vi "Parse State Queue++.vi"(0 "State Queue":string, 1 "Name(\"\" to use uuid)":string, 2 "Response Arguments":string, 7 "Error In (no error)":errorcluster, 9 "Dequeue Timeout(0ms)":i32, 11 "Response Timeout(5000ms)":i32=5000) -> (3 "Name Used":string, 4 "Remaining States":string, 6 "Current State":string, 8 "Arguments":string, 10 "Argument - State":string, 15 "From Who":string)   [LabVIEW 2014, in "JKI State Machine++.lvlib"]
doc: "Parses the JKI State Machine state queue and returns the current state that will execute next with the associated arguments.\n\n\n<b>Inputs:</b>\n - <b>State Queue</b>: The entire state queue is wired to this input. This should come from the main JKI State Machine shift register.\n - <b>Error In (no error)</b>: The error cluster from the JKI State Machine is wired to this input. If an error occures and appears on this input, the current state output returns the \"Error Handler\" state.\n - <b>Name(\"\" to use uuid)</b>: Module Name\n - If Input is \"\", an uuid will be used for module name. The module is marked as stand-alone mode and will not be included in module list.\n - Fi Input end with '#', the module will worked in worker mode. Modules with the same name will shared the same message queue. Any external message will be processed by one of the modules, depends on who is free.\n - Otherwise, the input string will be used as module name, which should be unique in system. JKISM will go to \"Critical Error\" state if duplicated module name is used in system.\n - <b>Response Timeout(5000ms)</b>: The timeout of waiting for response of sync-call from outside.\n - <b>Dequeue Timeout(0ms)</b>: The timeout of checking JKISM message queue.\n - <b>Response Arguments</b>: The response arguments from last state. It should come from the JKISM shift register.\n\n<b>Outputs:</b>\n - <b>Remaining States</b>: Returns all the next states that should execute after the current state completes. These should be passed through the current state in the state machine. These can also be modified or augmented within the current state if necessary.\n - <b>Arguments</b>: Returns any argument(s) that may be used in the current state string. These arguments come after the \">>\" characters. <b>Note:</b> The arguments variable must not contain any unprintable characters like linefeed or carriage return.\n - <b>Current State</b>: The state to be processed\n - <b>Name Used</b>: The actual name assigned to this JKISM module\n - <b>Argument - State</b>: If any core error occurs, this is the source state name\n - <b>From Who</b>: If <b>Current State</b> is called by ouside, this is the source JKISM module name."
uses:
  JKI State Machine++.lvlib
  _Support/Typedef/_Cross JKISM State Data.ctl
  _Support/Typedef/_JKISM_MSG_TYPE.ctl
  _Support/Typedef/_Cross JKISM State Response.ctl
  _Support/Typedef/_JKISM Status Change Event Data.ctl
  _Support/Typedef/_JKISM_GlobalLog_MSG.ctl
  _Support/Typedef/_JKISM_GlobalLog_MSG_TYPE.ctl
  _Support/JKISMQ/_Input Name to JKISM Mode.vi
  Utility/uuid.vi
  _Support/KeyWords.vi
  _Support/JKISMQ/_JKISMQFGV.vi
  _Support/FGV-BroadcastRegistry/FGV-BroadcastRegistry.vi
  _Support/FGV-BroadcastRegistry/global-Broadcast Cache Change Flag.vi
  <vilib>/regexp/Match Regular Expression.xnode
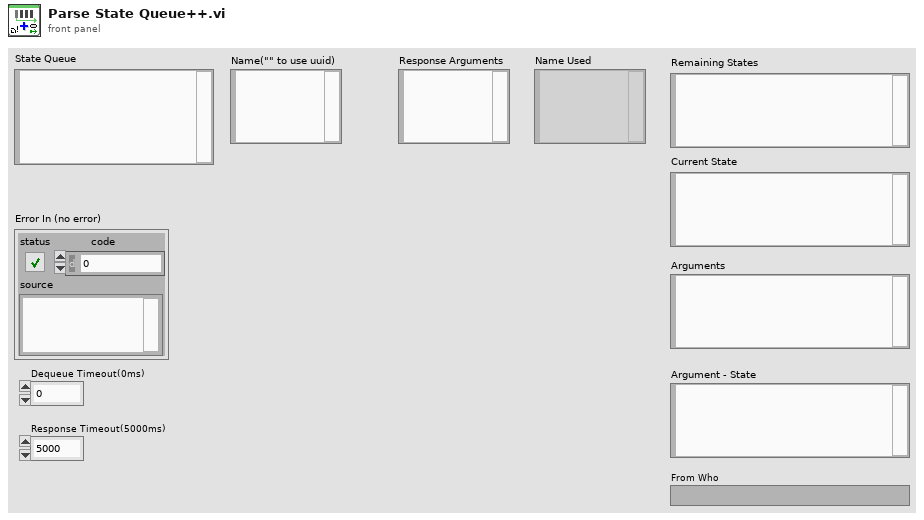
[diagram p1: front panel]
types:
  T1 = typedef "JKI State Machine++.lvlib/_JKISMQ.ctl" = cluster{"Module Name":string, "Queue":refnum<queue>, "Locked Status":refnum<data-value>, "Mode":T2, "User Event":refnum<user-event>, "Queue Count":i32, "Status Change Event":refnum<user-event>}
  T2 = typedef "JKI State Machine++.lvlib/_JKISM_MODE.ctl" = enum16{"Stand Alone", "JKISM", "Action Worker"}
  T3 = typedef "JKI State Machine++.lvlib/_JKISM_GlobalLog_MSG.ctl" = cluster{"Name(\"\" to use uuid)":string, "Current State":string, "Arguments":string, "Argument - State":string, "From Who":string, "Complete(T)/Start(F)":bool, "Type":T4}
  T4 = typedef "JKI State Machine++.lvlib/_JKISM_GlobalLog_MSG_TYPE.ctl" = enum16{"User Log", "State Change", "Status Change", "Register", "Unregister"}
  T5 = typedef "JKI State Machine++.lvlib/_JKISM_MSG_TYPE.ctl" = enum16{"Sync Message(-@)", "Async Message(->)", "Async without Response(->|)", "Async Response", "Broadcast(-><status>)", "Broadcast(-><interrupt>)", "Request to Post Message", "Request to Post Message without Reply", "Request to Publish Status"}
  T6 = typedef "JKI State Machine++.lvlib/_Cross JKISM State Data.ctl" = cluster{"Msg Type":T5, "state":string, "args":string, "source":string, "RespQ":refnum<queue>, "Pre-State":string, "Arg-State":string, "Target":string}
  T7 = typedef "JKI State Machine++.lvlib/_JKISM Status Change Event Data.ctl" = cluster{"ModuleName":string, "Status":string, "Arguments":string}
  T8 = typedef "JKI State Machine++.lvlib/_Cross JKISM State Response.ctl" = cluster{"error":errorcluster, "Response Data":string, "From Who":string}
  T9 = typedef "JKI State Machine++.lvlib/_JKISM_Broadcast_Response_Message_info.ctl" = cluster{"response message":string, "Priority":T10}
  T10 = typedef "JKI State Machine++.lvlib/JKISM++ Broadcast Message Type.ctl" = enum16{"Status", "Interrupt(High)"}
  T11 = cluster{"Target JKISM":string, "Target State":T9}[]
  T12 = typedef "JKI-State-Machine-Plus.lvlib/_Cross JKI StateMachine State Response.ctl" = cluster{"error":errorcluster, "Response Data":string, "From Who":string}
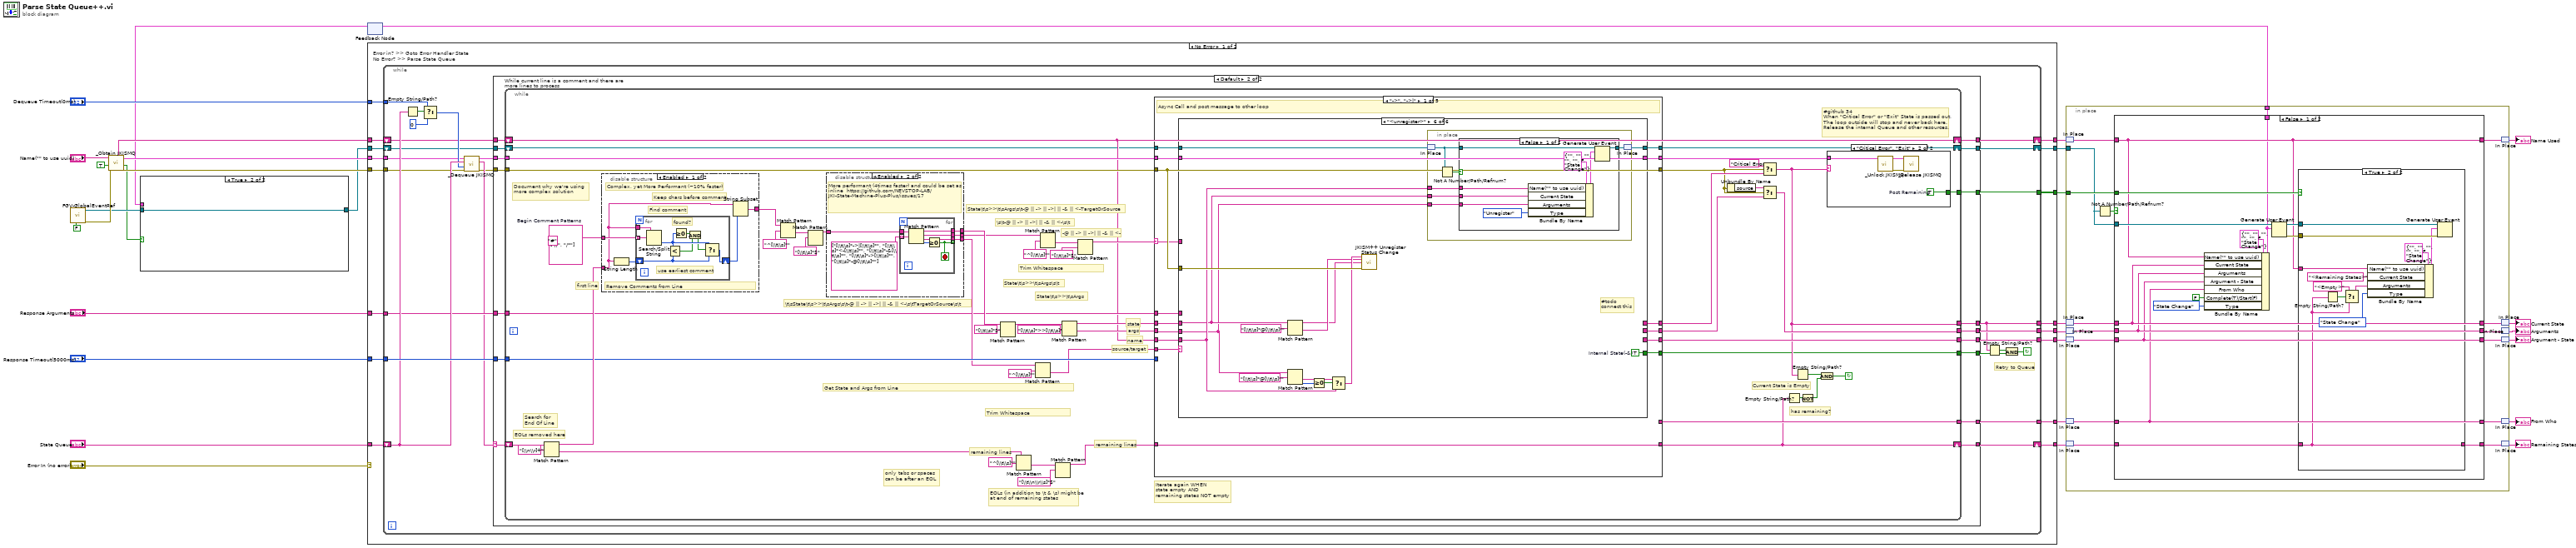
[diagram p0: block diagram]
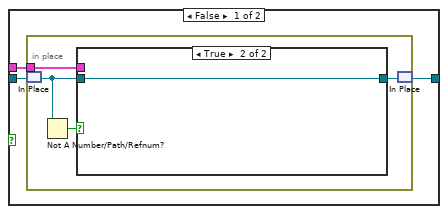
[diagram p2: hidden frame]
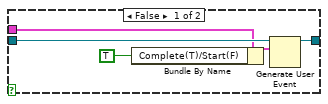
[diagram p3: hidden frame]
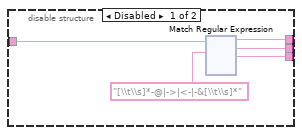
[diagram p7: hidden frame]
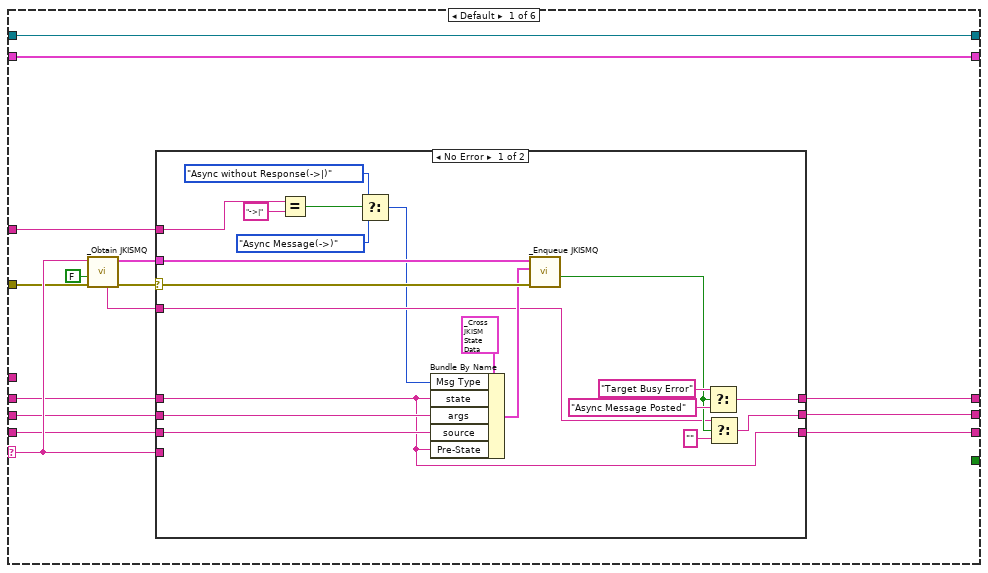
[diagram p9: hidden frame]
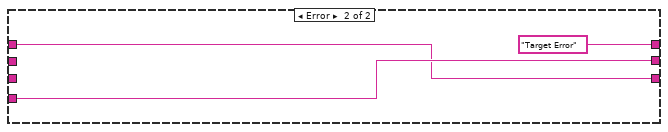
[diagram p10: hidden frame]
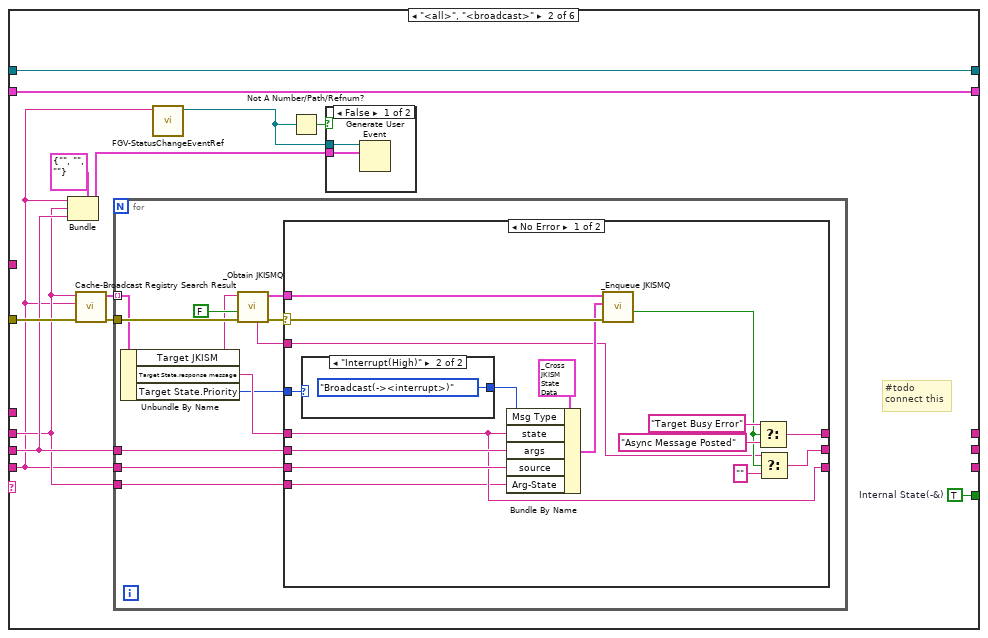
[diagram p11: hidden frame]
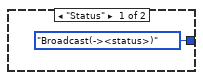
[diagram p13: hidden frame]
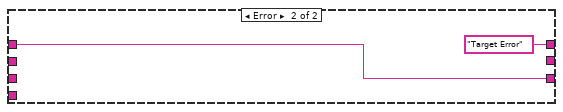
[diagram p14: hidden frame]
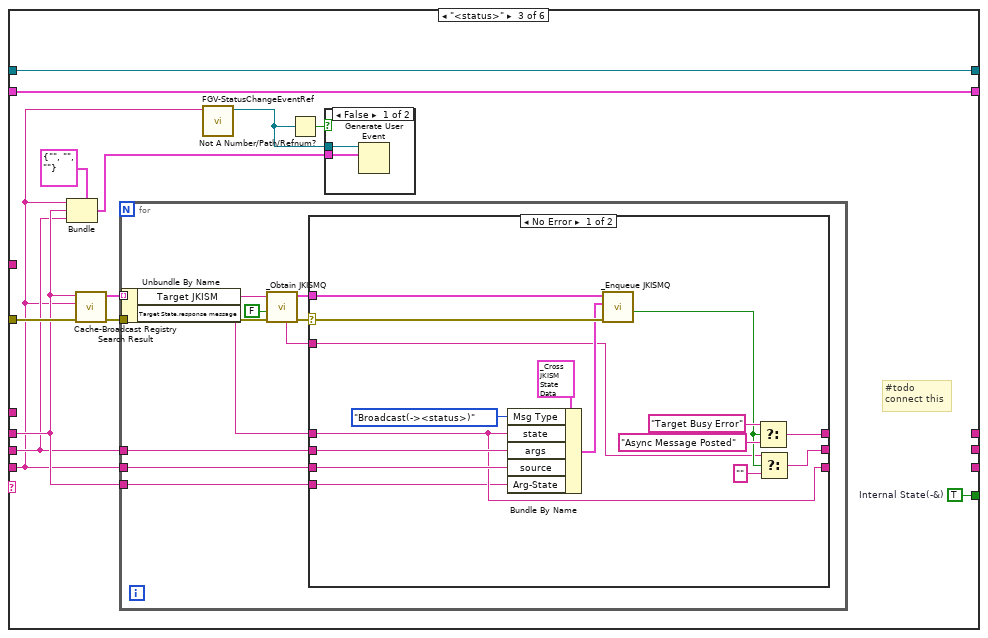
[diagram p15: hidden frame]
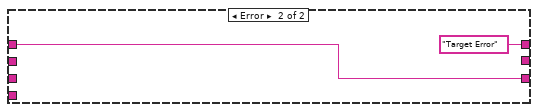
[diagram p17: hidden frame]
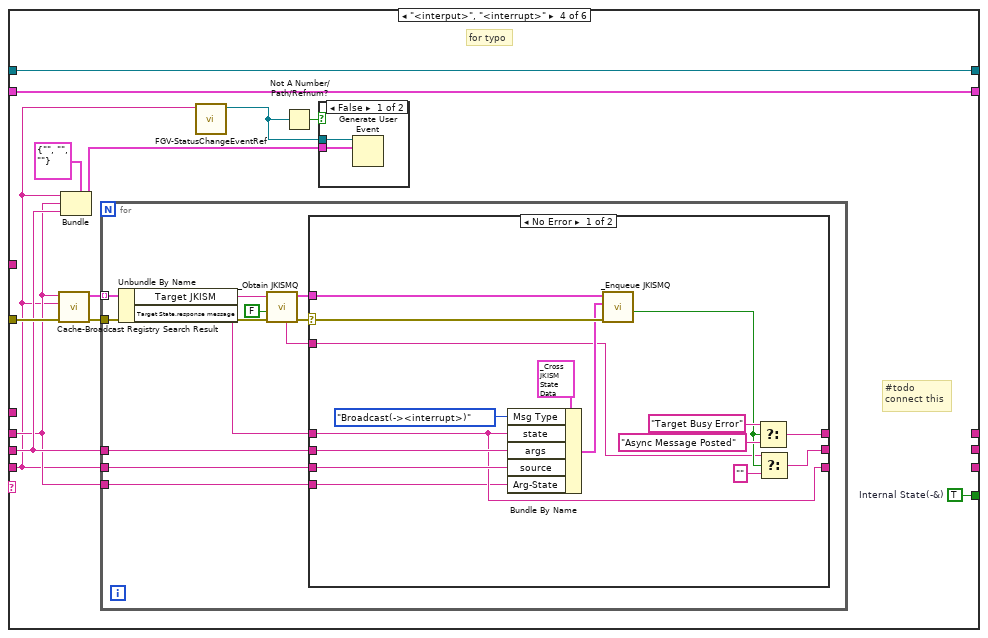
[diagram p18: hidden frame]
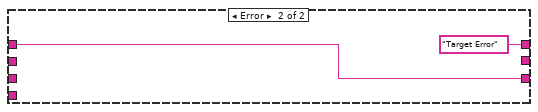
[diagram p20: hidden frame]
diagram:
  n1 = call "FGV-GlobalEventRef.vi"("Create(F)"=FALSE) -> ("error out"=w9:errorcluster, "JKISM Global Log Event"=w8:refnum<user-event>)  [unwired: 9 in]
  n2 = call "_Obtain JKISMQ.vi"("Error in"=w9, "create if not found? (T)"=TRUE, "Name(\"\" to use uuid) in"="Name(\"\" to use uuid)") -> ("Error out"=w25:errorcluster, "Create(T)/Cached(F)"=w4:bool, "JKISMQ"=w24:T1, "Name"=w3:string)  [unwired: 5 in]
  n3 = feedback #1() -> (w1:T3)  [unwired: 1 in]
  n4 = case shown="True" w4 {
    tunnel: w8 -> [w34 w45]
    tunnel: [w33 w45] -> w7
    tunnel: w1 -> [w32 _]
    frame False {
      n5 = in-place {
        in-place-border: w32 -> [w35]
        n6 = in-place-match #2(w34) -> (w37:refnum<user-event>)
        n7 = Not A Number/Path/Refnum?(number/path/refnum=w37) -> (NaN/Path/Refnum?=w38:bool)
        n8 = case shown="True" w38 {
          tunnel: w37 -> [w43 w44]
          tunnel: [w40 w44] -> w36
          tunnel: w35 -> [w39 _]
          frame False {
            n9 = Bundle By Name(cluster=w39, "Complete(T)/Start(F)"=TRUE) -> (w42:T3)
            n10 = Generate User Event(user event=w43, event data cluster=w42) -> (user event out=w40:refnum<user-event>)  [unwired: 2 in, 1 out]
          }
          frame True {
          }
        }
        n11 = in-place-match #2(w36) -> (w33:refnum<user-event>)
      }
    }
    frame True {
    }
  }
  n12 = case "Error in? >> Goto Error Handler State\nNo Error? >> Parse State Queue" shown="No Error" "Error In (no error)" {
    selector: "Error In (no error)" -> [_ w763]
    tunnel: [w59 w765] -> w13
    tunnel: [w61 "Error Handler"] -> w23
    tunnel: [w60 w759] -> w22
    tunnel: "State Queue" -> [w56 w765]
    tunnel: "Response Timeout(5000ms)" -> [w58 _]
    tunnel: w24 -> [w51 _]
    tunnel: [w57 _] -> w20
    tunnel: "Dequeue Timeout(0ms)" -> [w55 _]
    tunnel: [w54 _] -> w21
    tunnel: "Response Arguments" -> [w53 _]
    tunnel: w25 -> [w52 _]
    tunnel: w3 -> [w50 w757]
    tunnel: [w49 _] -> w14
    tunnel: w7 -> [w48 w756]
    tunnel: [w47 w757] -> w6
    tunnel: [w46 w756] -> w5
    frame No Error {
      n13 = while {
        tunnel: [w86] -> w60
        tunnel: w58 -> [w84]
        tunnel: [w83] -> w57
        tunnel: w55 -> [w79]
        tunnel: w52 -> [w74]
        tunnel: w51 -> [w73]
        shift-right: [w85] -> w59
        shift-left: w56 -> [w80]
        tunnel: w53 -> [w75]
        tunnel: [w67] -> w61
        tunnel: [w76] -> w54
        tunnel: [w65] -> w49
        shift-right: [w63] -> w47
        shift-left: w50 -> [w72]
        shift-right: [w62] -> w46
        shift-left: w48 -> [w64]
        stop <- w69 continue-if-true
        # "Retry to Queue"
        n14 = Empty String/Path?(string/path=w80) -> (empty?=w81:bool)
        n15 = Select(t=w79, s=w81, f=0) -> (s? t:f=w77:i32)
        n16 = call "_Dequeue JKISMQ.vi"("Error in"=w74, "Dequeue Timeout(0ms)"=w77, "State(s) in (\"\")"=w80, "JKISMQ in"=w73) -> ("Error out"=w70:errorcluster, "States Out"=w71:string, "JKISMQ out"=w82:T1)  [unwired: 5 in]
        n17 = case shown="Default" w71 {
          selector: w71 -> [_ w98]
          tunnel: [_ w104] -> w67
          tunnel: [_ w103] -> w86
          tunnel: [_ w102] -> w85
          tunnel: w84 -> [_ w101]
          tunnel: [_ w100] -> w83
          tunnel: w72 -> [w88 w99]
          tunnel: w82 -> [_ w97]
          tunnel: w70 -> [_ w96]
          tunnel: [_ w95] -> w76
          tunnel: w75 -> [_ w94]
          tunnel: [_ w93] -> w68
          tunnel: [_ w92] -> w65
          tunnel: w64 -> [w87 w91]
          tunnel: [w88 w90] -> w63
          tunnel: [w87 w89] -> w62
          frame "" {
            # "Dispatch Mode\n1. Error will Occurred\n2. Add Macro: Exit\n3. The Queue will regenerated\n4. But it will go Through Macro: Exit\n5. After Exit(queue released), then another Worker will be triggered."
            # "Do Nothing if Empty String"
            # "<< Wiring into the Case Selector is much more performant than using \"Empty String/Path?\" primitive"
          }
          frame Default {
            n18 = while "While current line is a comment and there are more lines to process" {
              tunnel: [w115] -> w104
              tunnel: [w119] -> w103
              shift-right: [w108] -> w102
              shift-left: w98 -> [w153]
              tunnel: w101 -> [w147]
              tunnel: [w118] -> w100
              tunnel: w97 -> [w146]
              tunnel: w96 -> [w123]
              tunnel: [w125] -> w95
              tunnel: w94 -> [w124]
              tunnel: [w112] -> w93
              tunnel: [w110] -> w92
              shift-right: [w107] -> w90
              shift-left: w99 -> [w107]
              shift-right: [w105] -> w89
              shift-left: w91 -> [w106]
              stop <- w111 continue-if-true
              (unwired) "#"
              w152 = string[] ["//", "/*"]  # Begin Comment Patterns
              # "#github 34\nWhen \"Critical Error\" or \"Exit\" State is passed out,\nThe loop outside will stop and never back here.\nRelease the internal Queue and other resources."
              # "source/target"
              # "name"
              # "-@ || -> || ->| || -& || <-"
              # "\\s\\t-@ || -> || ->| || -& || <-\\s\\t"
              # "Trim Whitespace"
              # "State\\t\\s>>\\t\\sArgs"
              # "State\\t\\s>>\\t\\sArgs\\s\\t"
              # "Get State and Args from Line"
              # "State\\t\\s>>\\t\\sArgs\\s\\t-@ || -> || ->| || -& || <-TargetOrSource"
              # "\\t\\sState\\t\\s>>\\t\\sArgs\\s\\t-@ || -> || ->| || -& || <-\\s\\tTargetOrSource\\s\\t"
              # "remaining lines"
              # "EOLs (in addition to \\t & \\s) might be at end of remaining states"
              # "Trim Whitespace"
              # "only tabs or spaces can be after an EOL"
              # "remaining lines"
              # "Iterate again WHEN\nstate empty AND\nremaining states NOT empty"
              # "args"
              # "state"
              # "Document why we're using more complex solution"
              # "EOLs removed here"
              # "Current State is Empty"
              # "has remaining?"
              # "first line"
              # "Search for End Of Line"
              n19 = Match Pattern(string=w153, regular expression="[\\n\\r]+") -> (before substring=w150:string, after substring=w148:string)  [unwired: 1 in, 2 out]
              n20 = disable-structure "Diagram Disable Structure" shown="Enabled" {
                disable-tunnel: w152 -> [w741 w752]
                disable-tunnel: [w740 w751] -> w151
                disable-tunnel: w150 -> [w739 w750]
                frame Enabled {
                  # "Remove Comments from Line"
                  # "Complex, yet More Performant (~10% faster)"
                  # "Keep chars before comment"
                  # "Find comment"
                  n21 = String Length(string=w739) -> (length=w738:i32)
                  n22 = for {
                    tunnel: w741 -> [w746] mode=indexing
                    shift-right: [w748] -> w737
                    shift-left: w738 -> [w749]
                    tunnel: w739 -> [w747]
                    # "found?"
                    # "use earliest comment"
                    n23 = Search/Split String(string=w747, search string/char (-)=w746) -> (offset of match=w745:i32)  [unwired: 1 in, 2 out]
                    n24 = Less?(x=w745, y=w749) -> (x < y?=w743:bool)
                    n25 = Greater Or Equal To 0?(x=w745) -> (x >= 0?=w744:bool)
                    n26 = And(x=w744, y=w743) -> (x .and. y?=w742:bool)
                    n27 = Select(t=w745, s=w742, f=w749) -> (s? t:f=w748:i32)
                  }
                  n28 = String Subset(string=w739, length (rest)=w737) -> (substring=w740:string)  [unwired: 1 in]
                }
                frame Disabled {
                  # "Since we keep substring *before* match in shift register, we will always trim to earliest comment"
                  # "Simpler, Yet Less Performant (~10% slower)"
                  n29 = for "For Each Comment Specifier" {
                    tunnel: w752 -> [w754] mode=indexing
                    shift-right: [w753] -> w751
                    shift-left: w750 -> [w755]
                    # "Keep Text Before Comment"
                    n30 = Search/Split String(string=w755, search string/char (-)=w754) -> (substring before match=w753:string)  [unwired: 1 in, 2 out]
                  }
                }
              }
              n31 = Match Pattern(string=w151, regular expression="^[\\t\\s]*") -> (after substring=w139:string)  [unwired: 1 in, 3 out]
              n32 = Match Pattern(string=w139, regular expression="[\\t\\s]*$") -> (before substring=w126:string)  [unwired: 1 in, 3 out]
              n33 = disable-structure shown="Enabled" {
                disable-tunnel: [w160 w278] -> w137
                disable-tunnel: [w159 w277] -> w134
                disable-tunnel: [w158 w276] -> w127
                disable-tunnel: w126 -> [w157 w280]
                frame Disabled {
                  n34 = xnode "Match Regular Expression"("input string"=w157, "regular expression"="[\\t\\s]*-@|->|<-|-&[\\t\\s]*") -> ("before match"=w160:string, "whole match"=w159:string, "after match"=w158:string)  [unwired: 4 in, 2 out]
                }
                frame Enabled {
                  # "More performant (4times faster) and could be set as inline  https://github.com/NEVSTOP-LAB/JKI-State-Machine-Plus-Plus/issues/17"
                  n35 = for {
                    tunnel: w280 -> [w287]
                    tunnel: string[] ["[\\t\\s]*->|[\\t\\s]*", "[\\t\\s]*<-[\\t\\s]*", "[\\t\\s]*-&[\\t\\s]*", "[\\t\\s]*->[\\t\\s]*", "[\\t\\s]*-@[\\t\\s]*"] -> [w286] mode=indexing
                    tunnel: [w284] -> _ mode=indexing
                    tunnel: [w283] -> w278
                    tunnel: [w282] -> w277
                    tunnel: [w281] -> w276
                    stop <- w284 stop-if-true
                    n36 = Match Pattern(string=w287, regular expression=w286) -> (before substring=w283:string, match substring=w282:string, after substring=w281:string, offset past match=w285:i32)  [unwired: 1 in]
                    n37 = Greater Or Equal To 0?(x=w285) -> (x >= 0?=w284:bool)
                  }
                }
              }
              n38 = Match Pattern(string=w137, regular expression="[\\t\\s]*$") -> (before substring=w136:string)  [unwired: 1 in, 3 out]
              n39 = Match Pattern(string=w148, regular expression="^[\\t\\s]*") -> (after substring=w140:string)  [unwired: 1 in, 3 out]
              n40 = Match Pattern(string=w127, regular expression="^[\\t\\s]*") -> (after substring=w117:string)  [unwired: 1 in, 3 out]
              n41 = Match Pattern(string=w134, regular expression="^[\\t\\s]*") -> (after substring=w130:string)  [unwired: 1 in, 3 out]
              n42 = Match Pattern(string=w140, regular expression="[\\t\\n\\r\\s]*$") -> (before substring=w109:string)  [unwired: 1 in, 3 out]
              n43 = Match Pattern(string=w136, regular expression="[\\t\\s]*>>[\\t\\s]*") -> (before substring=w133:string, after substring=w132:string)  [unwired: 1 in, 2 out]
              n44 = Match Pattern(string=w130, regular expression="[\\t\\s]*$") -> (before substring=w129:string)  [unwired: 1 in, 3 out]
              n45 = case shown="\"->\", \"->|\"" w129 {
                selector: w129 -> [w296 _ _ _ _]
                tunnel: w133 -> [w304 w553 w601 w687 w736]
                tunnel: w132 -> [w303 w552 w606 w688 w735]
                tunnel: [w307 w559 w608 w687 w736] -> w122
                tunnel: [w306 w558 w607 w688 w735] -> w121
                tunnel: w107 -> [w302 w551 w600 _ _]
                tunnel: w117 -> [w305 w557 w598 w676 w732]
                tunnel: w147 -> [_ w560 _ _ _]
                tunnel: w146 -> [w294 w548 w605 w683 w733]
                tunnel: w109 -> [w297 w546 w592 w675 w731]
                tunnel: [w301 w550 w599 w677 _] -> w125
                tunnel: w124 -> [w299 _ w604 _ _]
                tunnel: w123 -> [w300 w549 w602 w682 w734]
                tunnel: [w300 w549 w603 w681 w734] -> w120
                tunnel: [_ w547 w594 w678 w732] -> w118
                tunnel: [w295 w548 w595 w680 w733] -> w116
                tunnel: [w298 _ w593 _ _] -> w112
                tunnel: [w297 w546 w592 w674 w731] -> w108
                tunnel: w106 -> [w293 w545 w591 w673 w730]
                tunnel: [w292 w545 w591 w673 w730] -> w105
                frame "->", "->|" {
                  # "Async Call and post message to other loop"
                  n46 = case shown="\"<unregister>\"" w305 {
                    selector: w305 -> [w319 _ _ _ _ _]
                    tunnel: [w322 _ _ _ _ _] -> w307
                    tunnel: [w321 _ _ _ _ _] -> w306
                    tunnel: w304 -> [w317 w349 w399 w441 w483 w515]
                    tunnel: w303 -> [w316 w350 w398 w442 w482 w514]
                    tunnel: w302 -> [w315 w347 w395 w439 w484 w516]
                    tunnel: [w313 _ _ _ _ _] -> w301
                    tunnel: w300 -> [w312 w358 w406 w450 w496 w526]
                    tunnel: w299 -> [_ _ _ _ _ _]
                    tunnel: [_ w355 w403 w447 w498 w529] -> w298
                    tunnel: w296 -> [w310 _ _ _ _ _]
                    tunnel: [w309 w351 w402 w443 w487 w519] -> w295
                    tunnel: w294 -> [w309 w351 w402 w443 w487 w519]
                    tunnel: [w308 w346 w394 w438 w485 w517] -> w292
                    tunnel: w293 -> [w308 w346 w394 w438 w486 w518]
                    frame Default {
                      n47 = call "_Obtain JKISMQ.vi"("Error in"=w312, "create if not found? (T)"=FALSE, "Name(\"\" to use uuid) in"=w319) -> ("Error out"=w318:errorcluster, "JKISMQ"=w311:T1, "Name"=w314:string)  [unwired: 5 in, 1 out]
                      n48 = case shown="No Error" w318 {
                        selector: w318 -> [w341 _]
                        tunnel: w311 -> [w342 _]
                        tunnel: [w334 "Target Error" ("before match")] -> w322
                        tunnel: [w330 w344] -> w321
                        tunnel: w319 -> [_ w344]
                        tunnel: w317 -> [w329 w343]
                        tunnel: w316 -> [w339 _]
                        tunnel: w315 -> [w338 _]
                        tunnel: w314 -> [w331 _]
                        tunnel: [w329 w343] -> w313
                        tunnel: w310 -> [w328 _]
                        frame No Error {
                          n49 = Equal?(x=w328, y="->|") -> (x = y?=w326:bool)
                          n50 = Select(t=_JKISM_MSG_TYPE."Async without Response(->|)" ("Msg Type"), s=w326, f=_JKISM_MSG_TYPE."Async Message(->)" ("Msg Type")) -> (s? t:f=w323:T5)
                          n51 = Bundle By Name(cluster=T6 {"Msg Type"=enum."Sync Message(-@)", "state"="", "args"="", "source"="", "RespQ"=refnum, "Pre-State"="", "Arg-State"="", "Target"=""} ("Cross JKI State Machine State"), "Msg Type"=w323, "state"=w329, "args"=w339, "source"=w338, "Pre-State"=w329) -> (w337:T6)
                          n52 = call "_Enqueue JKISMQ.vi"("Error in"=w341, "Data"=w337, "JKISMQ in"=w342) -> ("Target Busy Error"=w332:bool)  [unwired: 6 in, 2 out]
                          n53 = Select(t="Target Busy Error" ("f"), s=w332, f="Async Message Posted" ("before match")) -> (s? t:f=w334:string)
                          n54 = Select(t=w331, s=w332, f="" ("before match")) -> (s? t:f=w330:string)
                        }
                        frame Error {
                        }
                      }
                    }
                    frame "<all>", "<broadcast>" {
                      w355 = TRUE  # Internal State(-&)
                      # "#todo\nconnect this"
                      n55 = Bundle(cluster=T7 {"ModuleName"="", "Status"="", "Arguments"=""} ("event data"), "ModuleName"=w347, "Status"=w349, "Arguments"=w350) -> (w352:T7)
                      n56 = call "Cache-Broadcast Registry Search Result.vi"("error in (no error)"=w358, "JKISM Name"=w347, "Broadcast state"=w349) -> ("error out"=w357:errorcluster, "Array"=w356:T11)  [unwired: 7 in]
                      n57 = for {
                        tunnel: w357 -> [w368]
                        tunnel: w356 -> [w364] mode=indexing
                        tunnel: w350 -> [w367]
                        tunnel: w347 -> [w366]
                        tunnel: w349 -> [w365]
                        n58 = Unbundle By Name(w364) -> ("Target JKISM"=w363:string, "Target State.response message"=w362:string, "Target State.Priority"=w361:T10)
                        n59 = call "_Obtain JKISMQ.vi"("Error in"=w368, "create if not found? (T)"=FALSE, "Name(\"\" to use uuid) in"=w363) -> ("Error out"=w370:errorcluster, "JKISMQ"=w371:T1, "Name"=w369:string)  [unwired: 5 in, 1 out]
                        n60 = case shown="No Error" w370 {
                          selector: w370 -> [w388 _]
                          tunnel: w371 -> [w389 _]
                          tunnel: [w381 "Target Error" ("before match")] -> _
                          tunnel: [w377 _] -> _
                          tunnel: w362 -> [w376 w392]
                          tunnel: w367 -> [w386 _]
                          tunnel: w366 -> [w385 _]
                          tunnel: w369 -> [w378 _]
                          tunnel: [w376 w392] -> _
                          tunnel: w365 -> [w375 _]
                          tunnel: w361 -> [w373 _]
                          frame No Error {
                            n61 = case shown="\"Interrupt(High)\"" w373 {
                              tunnel: [_JKISM_MSG_TYPE."Broadcast(-><status>)" ("Msg Type") _JKISM_MSG_TYPE."Broadcast(-><interrupt>)" ("Msg Type")] -> w374
                              frame "Status" {
                              }
                              frame "Interrupt(High)" {
                              }
                            }
                            n62 = Bundle By Name(cluster=T6 {"Msg Type"=enum."Sync Message(-@)", "state"="", "args"="", "source"="", "RespQ"=refnum, "Pre-State"="", "Arg-State"="", "Target"=""} ("Cross JKI State Machine State"), "Msg Type"=w374, "state"=w376, "args"=w386, "source"=w385, "Arg-State"=w375) -> (w384:T6)
                            n63 = call "_Enqueue JKISMQ.vi"("Error in"=w388, "Data"=w384, "JKISMQ in"=w389) -> ("Target Busy Error"=w379:bool)  [unwired: 6 in, 2 out]
                            n64 = Select(t="Target Busy Error" ("f"), s=w379, f="Async Message Posted" ("before match")) -> (s? t:f=w381:string)
                            n65 = Select(t=w378, s=w379, f="" ("before match")) -> (s? t:f=w377:string)
                          }
                          frame Error {
                          }
                        }
                      }
                      n66 = call "FGV-StatusChangeEventRef.vi"("Name(\"\" to use uuid) in"=w347) -> ("Status Change Event"=w348:refnum<user-event>)  [unwired: 9 in, 1 out]
                      n67 = Not A Number/Path/Refnum?(number/path/refnum=w348) -> (NaN/Path/Refnum?=w354:bool)
                      n68 = case shown="False" w354 {
                        tunnel: w348 -> [w360 _]
                        tunnel: w352 -> [w359 _]
                        frame False {
                          n69 = Generate User Event(user event=w360, event data cluster=w359) -> ()  [unwired: 2 in, 2 out]
                        }
                        frame True {
                        }
                      }
                    }
                    frame "<status>" {
                      w403 = TRUE  # Internal State(-&)
                      # "#todo\nconnect this"
                      n70 = Bundle(cluster=T7 {"ModuleName"="", "Status"="", "Arguments"=""} ("event data"), "ModuleName"=w395, "Status"=w399, "Arguments"=w398) -> (w397:T7)
                      n71 = call "Cache-Broadcast Registry Search Result.vi"("error in (no error)"=w406, "JKISM Name"=w395, "Broadcast state"=w399) -> ("error out"=w405:errorcluster, "Array"=w404:T11)  [unwired: 7 in]
                      n72 = for {
                        tunnel: w405 -> [w415]
                        tunnel: w404 -> [w411] mode=indexing
                        tunnel: w398 -> [w414]
                        tunnel: w395 -> [w413]
                        tunnel: w399 -> [w412]
                        n73 = Unbundle By Name(w411) -> ("Target JKISM"=w410:string, "Target State.response message"=w409:string)
                        n74 = call "_Obtain JKISMQ.vi"("Error in"=w415, "create if not found? (T)"=FALSE, "Name(\"\" to use uuid) in"=w410) -> ("Error out"=w417:errorcluster, "JKISMQ"=w418:T1, "Name"=w416:string)  [unwired: 5 in, 1 out]
                        n75 = case shown="No Error" w417 {
                          selector: w417 -> [w434 _]
                          tunnel: w418 -> [w435 _]
                          tunnel: [w427 "Target Error" ("before match")] -> _
                          tunnel: [w423 _] -> _
                          tunnel: w409 -> [w422 w436]
                          tunnel: w414 -> [w432 _]
                          tunnel: w413 -> [w431 _]
                          tunnel: w416 -> [w424 _]
                          tunnel: [w422 w436] -> _
                          tunnel: w412 -> [w421 _]
                          frame No Error {
                            n76 = Bundle By Name(cluster=T6 {"Msg Type"=enum."Sync Message(-@)", "state"="", "args"="", "source"="", "RespQ"=refnum, "Pre-State"="", "Arg-State"="", "Target"=""} ("Cross JKI State Machine State"), "Msg Type"=_JKISM_MSG_TYPE."Broadcast(-><status>)", "state"=w422, "args"=w432, "source"=w431, "Arg-State"=w421) -> (w430:T6)
                            n77 = call "_Enqueue JKISMQ.vi"("Error in"=w434, "Data"=w430, "JKISMQ in"=w435) -> ("Target Busy Error"=w425:bool)  [unwired: 6 in, 2 out]
                            n78 = Select(t="Target Busy Error" ("f"), s=w425, f="Async Message Posted" ("before match")) -> (s? t:f=w427:string)
                            n79 = Select(t=w424, s=w425, f="" ("before match")) -> (s? t:f=w423:string)
                          }
                          frame Error {
                          }
                        }
                      }
                      n80 = call "FGV-StatusChangeEventRef.vi"("Name(\"\" to use uuid) in"=w395) -> ("Status Change Event"=w396:refnum<user-event>)  [unwired: 9 in, 1 out]
                      n81 = Not A Number/Path/Refnum?(number/path/refnum=w396) -> (NaN/Path/Refnum?=w401:bool)
                      n82 = case shown="False" w401 {
                        tunnel: w396 -> [w408 _]
                        tunnel: w397 -> [w407 _]
                        frame False {
                          n83 = Generate User Event(user event=w408, event data cluster=w407) -> ()  [unwired: 2 in, 2 out]
                        }
                        frame True {
                        }
                      }
                    }
                    frame "<interput>", "<interrupt>" {
                      w447 = TRUE  # Internal State(-&)
                      # "for typo"
                      # "#todo\nconnect this"
                      n84 = call "Cache-Broadcast Registry Search Result.vi"("error in (no error)"=w450, "JKISM Name"=w439, "Broadcast state"=w441) -> ("error out"=w449:errorcluster, "Array"=w448:T11)  [unwired: 7 in]
                      n85 = Bundle(cluster=T7 {"ModuleName"="", "Status"="", "Arguments"=""} ("event data"), "ModuleName"=w439, "Status"=w441, "Arguments"=w442) -> (w444:T7)
                      n86 = for {
                        tunnel: w449 -> [w459]
                        tunnel: w448 -> [w455] mode=indexing
                        tunnel: w442 -> [w458]
                        tunnel: w439 -> [w457]
                        tunnel: w441 -> [w456]
                        n87 = Unbundle By Name(w455) -> ("Target JKISM"=w454:string, "Target State.response message"=w453:string)
                        n88 = call "_Obtain JKISMQ.vi"("Error in"=w459, "create if not found? (T)"=FALSE, "Name(\"\" to use uuid) in"=w454) -> ("Error out"=w461:errorcluster, "JKISMQ"=w462:T1, "Name"=w460:string)  [unwired: 5 in, 1 out]
                        n89 = case shown="No Error" w461 {
                          selector: w461 -> [w478 _]
                          tunnel: w462 -> [w479 _]
                          tunnel: [w471 "Target Error" ("before match")] -> _
                          tunnel: [w467 _] -> _
                          tunnel: w453 -> [w466 w480]
                          tunnel: w458 -> [w476 _]
                          tunnel: w457 -> [w475 _]
                          tunnel: w460 -> [w468 _]
                          tunnel: [w466 w480] -> _
                          tunnel: w456 -> [w465 _]
                          frame No Error {
                            n90 = Bundle By Name(cluster=T6 {"Msg Type"=enum."Sync Message(-@)", "state"="", "args"="", "source"="", "RespQ"=refnum, "Pre-State"="", "Arg-State"="", "Target"=""} ("Cross JKI State Machine State"), "Msg Type"=_JKISM_MSG_TYPE."Broadcast(-><interrupt>)", "state"=w466, "args"=w476, "source"=w475, "Arg-State"=w465) -> (w474:T6)
                            n91 = call "_Enqueue JKISMQ.vi"("Error in"=w478, "Data"=w474, "JKISMQ in"=w479) -> ("Target Busy Error"=w469:bool)  [unwired: 6 in, 2 out]
                            n92 = Select(t="Target Busy Error" ("f"), s=w469, f="Async Message Posted" ("before match")) -> (s? t:f=w471:string)
                            n93 = Select(t=w468, s=w469, f="" ("before match")) -> (s? t:f=w467:string)
                          }
                          frame Error {
                          }
                        }
                      }
                      n94 = call "FGV-StatusChangeEventRef.vi"("Name(\"\" to use uuid) in"=w439) -> ("Status Change Event"=w440:refnum<user-event>)  [unwired: 9 in, 1 out]
                      n95 = Not A Number/Path/Refnum?(number/path/refnum=w440) -> (NaN/Path/Refnum?=w446:bool)
                      n96 = case shown="False" w446 {
                        tunnel: w440 -> [w452 _]
                        tunnel: w444 -> [w451 _]
                        frame False {
                          n97 = Generate User Event(user event=w452, event data cluster=w451) -> ()  [unwired: 2 in, 2 out]
                        }
                        frame True {
                        }
                      }
                    }
                    frame "<register>" {
                      w498 = TRUE  # Internal State(-&)
                      # "#todo\nconnect this"
                      n98 = Match Pattern(string=w483, regular expression="[\\t\\s]*@[\\t\\s]*") -> (before substring=w489:string, after substring=w490:string)  [unwired: 1 in, 2 out]
                      n99 = Match Pattern(string=w482, regular expression="[\\t\\s]*@[\\t\\s]*") -> (before substring=w488:string, after substring=w491:string, offset past match=w494:i32)  [unwired: 1 in, 1 out]
                      n100 = Greater Or Equal To 0?(x=w494) -> (x >= 0?=w493:bool)
                      n101 = Select(t=w491, s=w493, f=w484) -> (s? t:f=w492:string)
                      n102 = call "JKISM++ Register Status Change.vi"("JKISM Name"=w492, "Source JKISM Name (* as Default)"=w490, "Status"=w489, "Response Message (if \"\", same as Source Message)"=w488, "Error in"=w496) -> ()  [unwired: 9 in, 2 out]
                      n103 = in-place {
                        in-place-border: w484 -> [w501]
                        in-place-border: w483 -> [w500]
                        in-place-border: w482 -> [w499]
                        n104 = in-place-match #3(w486) -> (w503:refnum<user-event>)
                        n105 = Not A Number/Path/Refnum?(number/path/refnum=w503) -> (NaN/Path/Refnum?=w504:bool)
                        n106 = case shown="True" w504 {
                          tunnel: w503 -> [w512 w513]
                          tunnel: w501 -> [w509 _]
                          tunnel: [w508 w513] -> w502
                          tunnel: w500 -> [w506 _]
                          tunnel: w499 -> [w505 _]
                          frame False {
                            n107 = Bundle By Name(cluster=T3 {"Name(\"\" to use uuid)"="", "Current State"="", "Arguments"="", "Argument - State"="", "From Who"="", "Complete(T)/Start(F)"=FALSE, "Type"=enum."State Change"} ("event data"), "Name(\"\" to use uuid)"=w509, "Current State"=w506, "Arguments"=w505, "Type"=_JKISM_GlobalLog_MSG_TYPE."Register") -> (w510:T3)
                            n108 = Generate User Event(user event=w512, event data cluster=w510) -> (user event out=w508:refnum<user-event>)  [unwired: 2 in, 1 out]
                          }
                          frame True {
                          }
                        }
                        n109 = in-place-match #3(w502) -> (w485:refnum<user-event>)
                      }
                    }
                    frame "<unregister>" {
                      w529 = TRUE  # Internal State(-&)
                      # "#todo\nconnect this"
                      n110 = Match Pattern(string=w515, regular expression="[\\t\\s]*@[\\t\\s]*") -> (before substring=w520:string, after substring=w521:string)  [unwired: 1 in, 2 out]
                      n111 = Match Pattern(string=w514, regular expression="[\\t\\s]*@[\\t\\s]*") -> (after substring=w523:string, offset past match=w525:i32)  [unwired: 1 in, 2 out]
                      n112 = Greater Or Equal To 0?(x=w525) -> (x >= 0?=w524:bool)
                      n113 = Select(t=w523, s=w524, f=w516) -> (s? t:f=w522:string)
                      n114 = call "JKISM++ Unregister Status Change.vi"("JKISM Name"=w522, "Source JKISM Name"=w521, "Status"=w520, "Error in"=w526) -> ()  [unwired: 10 in, 2 out]
                      n115 = in-place {
                        in-place-border: w516 -> [w532]
                        in-place-border: w515 -> [w531]
                        in-place-border: w514 -> [w530]
                        n116 = in-place-match #4(w518) -> (w534:refnum<user-event>)
                        n117 = Not A Number/Path/Refnum?(number/path/refnum=w534) -> (NaN/Path/Refnum?=w535:bool)
                        n118 = case shown="False" w535 {
                          tunnel: w534 -> [w543 w544]
                          tunnel: w532 -> [w540 _]
                          tunnel: [w539 w544] -> w533
                          tunnel: w531 -> [w537 _]
                          tunnel: w530 -> [w536 _]
                          frame False {
                            n119 = Bundle By Name(cluster=T3 {"Name(\"\" to use uuid)"="", "Current State"="", "Arguments"="", "Argument - State"="", "From Who"="", "Complete(T)/Start(F)"=FALSE, "Type"=enum."State Change"} ("event data"), "Name(\"\" to use uuid)"=w540, "Current State"=w537, "Arguments"=w536, "Type"=_JKISM_GlobalLog_MSG_TYPE."Unregister") -> (w541:T3)
                            n120 = Generate User Event(user event=w543, event data cluster=w541) -> (user event out=w539:refnum<user-event>)  [unwired: 2 in, 1 out]
                          }
                          frame True {
                          }
                        }
                        n121 = in-place-match #4(w533) -> (w517:refnum<user-event>)
                      }
                    }
                  }
                }
                frame "-@" {
                  # "Synchonized Call send msg and wait response"
                  n122 = call "_Obtain JKISMQ.vi"("Error in"=w549, "create if not found? (T)"=FALSE, "Name(\"\" to use uuid) in"=w557) -> ("Error out"=w555:errorcluster, "JKISMQ"=w556:T1)  [unwired: 5 in, 2 out]
                  n123 = case shown="No Error" w555 {
                    selector: w555 -> [w578 _]
                    tunnel: w560 -> [w586 _]
                    tunnel: w556 -> [w587 _]
                    tunnel: [FALSE _] -> _
                    tunnel: [w585 "Target Error" ("before match")] -> w559
                    tunnel: [w570 w588] -> w558
                    tunnel: w557 -> [w564 w588]
                    tunnel: w553 -> [w565 w589]
                    tunnel: w552 -> [w566 _]
                    tunnel: w551 -> [w567 _]
                    tunnel: [w565 w589] -> w550
                    tunnel: [w561 w588] -> w547
                    frame No Error {
                      n124 = call "_Create Resp Queue.vi"("max queue size (-1, unlimited)"=1, "error in (no error)"=w578) -> ("error out"=w574:errorcluster, "queue out"=w569:refnum<queue>)  [unwired: 7 in, 1 out]
                      n125 = Bundle By Name(cluster=T6 {"Msg Type"=enum."Sync Message(-@)", "state"="", "args"="", "source"="", "RespQ"=refnum, "Pre-State"="", "Arg-State"="", "Target"=""} ("Cross JKI State Machine State"), "Msg Type"=_JKISM_MSG_TYPE."Sync Message(-@)", "state"=w565, "args"=w566, "source"=w567, "RespQ"=w569, "Pre-State"=w565) -> (w579:T6)
                      n126 = call "_Enqueue JKISMQ.vi"("Error in"=w574, "Data"=w579, "JKISMQ in"=w587) -> ("Error out"=w575:errorcluster)  [unwired: 6 in, 2 out]
                      n127 = Dequeue Element(queue=w569, timeout in ms (-1)=w586, error in (no error)=w575) -> (queue out=w577:refnum<queue>, element=w573:T12, timed out?=w584:bool, error out=w576:errorcluster)
                      n128 = Unbundle(w573) -> ("Response Data"=w571:string, "From Who"=w562:string)  [unwired: 1 out]
                      n129 = Not(x=w584) -> (.not. x?=w563:bool)
                      n130 = Release Queue(queue=w577, error in (no error)=w576) -> ()  [unwired: 1 in, 3 out]
                      n131 = Select(t=w571, s=w563, f=w564) -> (s? t:f=w570:string)
                      n132 = Select(t="Response" ("f"), s=w563, f="Target Timeout Error" ("before match")) -> (s? t:f=w585:string)
                      n133 = Select(t=w562, s=w563, f=w564) -> (s? t:f=w561:string)
                    }
                    frame Error {
                    }
                  }
                }
                frame "-&" {
                  w593 = TRUE  # Internal State(-&)
                  # "Synchonized Call send msg and wait response"
                  n134 = call "_Unlock JKISMQ.vi"("Error in"=w602, "JKISMQ in"=w605) -> ("Error out"=w603:errorcluster, "JKISMQ out"=w595:T1)  [unwired: 8 in]
                  n135 = Match Pattern(string=w598, regular expression="[\\t\\s]*>>>>[\\t\\s]*") -> (before substring=w594:string, after substring=w596:string)  [unwired: 1 in, 2 out]
                  n136 = case shown="\"PostPostMsg\"" w601 {
                    selector: w601 -> [w609 _ _]
                    tunnel: ["Critical Error" ("before match") w617 w659] -> w608
                    tunnel: [w611 w618 w658] -> w607
                    tunnel: w594 -> [_ w615 w648]
                    tunnel: w606 -> [_ _ w651]
                    tunnel: w604 -> [_ w621 w650]
                    tunnel: w602 -> [_ w622 w649]
                    tunnel: w600 -> [_ w619 w646]
                    tunnel: [_ w616 w647] -> w599
                    tunnel: w596 -> [_ w614 w647]
                    frame Default {
                      n137 = Concatenate Strings("Framework error, it recieved \"" ("before match"), w609, "\" which is not expected." ("before match")) -> (w611:string)
                    }
                    frame "PostPostMsg" {
                      n138 = call "_Obtain JKISMQ.vi"("Error in"=w622, "create if not found? (T)"=FALSE, "Name(\"\" to use uuid) in"=w615) -> ("Error out"=w624:errorcluster, "JKISMQ"=w625:T1, "Name"=w623:string)  [unwired: 5 in, 1 out]
                      n139 = case shown="No Error" w624 {
                        selector: w624 -> [w641 _]
                        tunnel: w625 -> [w642 _]
                        tunnel: [w634 "Target Error" ("before match")] -> w617
                        tunnel: [w629 w644] -> w618
                        tunnel: w615 -> [_ w644]
                        tunnel: "Async Response" ("Response Arguments") -> [w631 w643]
                        tunnel: w621 -> [w639 _]
                        tunnel: w619 -> [w638 _]
                        tunnel: w623 -> [w632 _]
                        tunnel: [w628 w643] -> w616
                        tunnel: w614 -> [w628 _]
                        frame No Error {
                          n140 = Bundle By Name(cluster=T6 {"Msg Type"=enum."Sync Message(-@)", "state"="", "args"="", "source"="", "RespQ"=refnum, "Pre-State"="", "Arg-State"="", "Target"=""} ("Cross JKI State Machine State"), "Msg Type"=_JKISM_MSG_TYPE."Async Response", "state"=w631, "args"=w639, "source"=w638, "Pre-State"=w628) -> (w637:T6)
                          n141 = call "_Enqueue JKISMQ.vi"("Error in"=w641, "Data"=w637, "JKISMQ in"=w642) -> ("Target Busy Error"=w630:bool)  [unwired: 6 in, 2 out]
                          n142 = Select(t="Target Busy Error" ("f"), s=w630, f="" ("before match")) -> (s? t:f=w634:string)
                          n143 = Select(t=w632, s=w630, f="" ("before match")) -> (s? t:f=w629:string)
                        }
                        frame Error {
                        }
                      }
                    }
                    frame "PostSendMsg" {
                      n144 = Obtain Queue(name (unnamed)=w651, element data type=T8 {"error"={"status"=FALSE, "code"=0, "source"=""}, "Response Data"="", "From Who"=""} ("Cross JKI State Machine Response"), create if not found? (T)=FALSE, error in (no error)=w649) -> (queue out=w655:refnum<queue>, error out=w654:errorcluster)  [unwired: 1 in, 1 out]
                      n145 = case shown="No Error" w654 {
                        selector: w654 -> [w666 w670]
                        tunnel: [_ "Target Error" ("before match")] -> w659
                        tunnel: [_ w669] -> w658
                        tunnel: w655 -> [w668 w671]
                        tunnel: [w667 w671] -> w657
                        tunnel: [w665 w670] -> w656
                        tunnel: w648 -> [_ w669]
                        tunnel: w650 -> [w662 _]
                        tunnel: w646 -> [w660 _]
                        frame No Error {
                          n146 = Bundle(cluster=T8 {"error"={"status"=FALSE, "code"=0, "source"=""}, "Response Data"="", "From Who"=""} ("element"), "error"=errorcluster {"status"=FALSE, "code"=0, "source"=""}, "Response Data"=w662, "From Who"=w660) -> (w663:T8)
                          n147 = Enqueue Element(queue=w668, element=w663, error in (no error)=w666) -> (queue out=w667:refnum<queue>, error out=w665:errorcluster)  [unwired: 1 in, 1 out]
                        }
                        frame Error {
                        }
                      }
                      n148 = Release Queue(queue=w657, error in (no error)=w656) -> ()  [unwired: 1 in, 3 out]
                    }
                  }
                }
                frame "", "<-" {
                  # "\"<-\"  : Added by Other JKI State Loop |  \"\" : Added by Current Loop"
                  n149 = Match Pattern(string=w676, regular expression="[\\t\\s]*>>>>[\\t\\s]*") -> (before substring=w678:string, after substring=w677:string)  [unwired: 1 in, 2 out]
                  n150 = To Lower Case(string=w687) -> (all lower case string=w686:string)
                  n151 = Equal?(x=w686, y="exit") -> (x = y?=w684:bool)
                  n152 = case shown="True" w684 {
                    tunnel: w675 -> [w689 w692]
                    tunnel: w683 -> [w690 w699]
                    tunnel: w682 -> [w691 w697]
                    tunnel: [w691 w695] -> w681
                    tunnel: [w690 w694] -> w680
                    tunnel: [w689 w693] -> w674
                    frame False {
                    }
                    frame True {
                      n153 = call "_Lock State JKISMQ.vi"("Error in"=w697, "JKISMQ in"=w699) -> ("Error out"=w696:errorcluster, "lock"=w698:bool, "JKISMQ out"=w694:T1)  [unwired: 7 in]
                      n154 = case shown="True" w698 {
                        tunnel: w692 -> [_ w716]
                        tunnel: w696 -> [w701 w707]
                        tunnel: [w701 w707] -> w695
                        tunnel: [w700 w705] -> w693
                        tunnel: w692 -> [w700 _]
                        frame False {
                        }
                        frame True {
                          # "#NOTE\nSync Call Post Exit , need to response."
                          n155 = Match Pattern(string=w716, regular expression="PostSendMsg >>") -> (before substring=w706:string, after substring=w713:string)  [unwired: 1 in, 2 out]
                          n156 = Match Pattern(string=w713, regular expression="-&") -> (before substring=w709:string, after substring=w703:string)  [unwired: 1 in, 2 out]
                          n157 = Match Pattern(string=w709, regular expression="^[\\t\\s]*") -> (after substring=w712:string)  [unwired: 1 in, 3 out]
                          n158 = Match Pattern(string=w712, regular expression="[\\t\\s]*$") -> (before substring=w708:string)  [unwired: 1 in, 3 out]
                          n159 = Match Pattern(string=w703, regular expression="[\\n\\r]") -> (after substring=w702:string)  [unwired: 1 in, 3 out]
                          n160 = Obtain Queue(name (unnamed)=w708, element data type=T8 {"error"={"status"=FALSE, "code"=0, "source"=""}, "Response Data"="", "From Who"=""} ("Cross JKI State Machine Response"), create if not found? (T)=FALSE, error in (no error)=w707) -> (queue out=w721:refnum<queue>, error out=w722:errorcluster)  [unwired: 1 in, 1 out]
                          n161 = Concatenate Strings(w706, w702) -> (w705:string)
                          n162 = case shown="No Error" w722 {
                            selector: w722 -> [w725 w728]
                            tunnel: w721 -> [w727 w729]
                            tunnel: [w726 w729] -> w719
                            tunnel: [w724 w728] -> w720
                            frame No Error {
                              n163 = Enqueue Element(queue=w727, element=T8 {"error"={"status"=FALSE, "code"=0, "source"=""}, "Response Data"="", "From Who"=""}, error in (no error)=w725) -> (queue out=w726:refnum<queue>, error out=w724:errorcluster)  [unwired: 1 in, 1 out]
                            }
                            frame Error {
                            }
                          }
                          n164 = Release Queue(queue=w719, error in (no error)=w720) -> ()  [unwired: 1 in, 3 out]
                        }
                      }
                    }
                  }
                }
                frame Default {
                  # "Error, should not be here."
                }
              }
              n165 = Unbundle By Name(w120) -> ("source"=w114:string)
              n166 = Select(t="Critical Error", s=w120, f=w122) -> (s? t:f=w115:string)
              n167 = Select(t=w114, s=w120, f=w121) -> (s? t:f=w119:string)
              n168 = Empty String/Path?(string/path=w108) -> (empty?=w155:bool)
              n169 = Empty String/Path?(string/path=w115) -> (empty?=w156:bool)
              n170 = Not(x=w155) -> (.not. x?=w149:bool)
              n171 = And(x=w156, y=w149) -> (x .and. y?=w111:bool)
              n172 = case shown="\"Critical Error\", \"Exit\"" w115 {
                tunnel: w116 -> [_ w291]
                tunnel: [_ w289] -> w110
                frame "False", Default {
                }
                frame "Critical Error", "Exit" {
                  w289 = TRUE  # Post Remaining
                  n173 = call "_Unlock JKISMQ.vi"("JKISMQ in"=w291) -> ("Error out"=w288:errorcluster, "JKISMQ out"=w290:T1)  [unwired: 9 in]
                  n174 = call "_Release JKISMQ.vi"("Error in"=w288, "JKISMQ"=w290) -> ()  [unwired: 9 in, 1 out]
                }
              }
            }
          }
        }
        n175 = Empty String/Path?(string/path=w67) -> (empty?=w66:bool)
        n176 = And(x=w66, y=w68) -> (x .and. y?=w69:bool)
      }
    }
    frame Error {
      # "Goto Error Handler State >>"
      # "preserve remaining states >>"
      n177 = Unbundle By Name(w763) -> ("code"=w761:i32, "source"=w762:string)
      n178 = call "JKISM++ Make String Arguments Safe.vi"("Argurment String"=w762) -> ("Safe Argurment String"=w760:string)  [unwired: 8 in]
      n179 = Format Into String(format string="[Code: %d]%s", w761, w760) -> (resulting string=w759:string)  [unwired: 2 in, 1 out]
    }
  }
  n180 = in-place {
    in-place-border: w14 -> [w770]
    in-place-border: w5 -> [w767]
    in-place-border: [w766] -> w2
    n181 = in-place-match #5(w6) -> (w776:string)
    n182 = in-place-match #6(w23) -> (w778:string)
    n183 = in-place-match #7(w22) -> (w779:string)
    n184 = in-place-match #8(w21) -> (w780:string)
    n185 = in-place-match #9(w20) -> (w777:string)
    n186 = in-place-match #10(w13) -> (w768:string)
    n187 = Not A Number/Path/Refnum?(number/path/refnum=w767) -> (NaN/Path/Refnum?=w781:bool)
    n188 = case shown="False" w781 {
      tunnel: w767 -> [w796 _]
      tunnel: w778 -> [w795 w814]
      tunnel: [w795 w814] -> w775
      tunnel: w779 -> [w794 w813]
      tunnel: [w794 w813] -> w774
      tunnel: [w793 w812] -> w773
      tunnel: w780 -> [w793 w812]
      tunnel: [w792 w811] -> w772
      tunnel: w777 -> [w792 w811]
      tunnel: w776 -> [w784 w810]
      tunnel: [w784 w810] -> w771
      tunnel: w770 -> [w786 _]
      tunnel: [w785 w809] -> w769
      tunnel: w768 -> [w787 w809]
      tunnel: [w782 _] -> w766
      frame False {
        n189 = Bundle By Name(cluster=T3 {"Name(\"\" to use uuid)"="", "Current State"="", "Arguments"="", "Argument - State"="", "From Who"="", "Complete(T)/Start(F)"=FALSE, "Type"=enum."State Change"} ("event data"), "Name(\"\" to use uuid)"=w784, "Current State"=w795, "Arguments"=w794, "Argument - State"=w793, "From Who"=w792, "Complete(T)/Start(F)"=FALSE, "Type"=_JKISM_GlobalLog_MSG_TYPE."State Change") -> (w782:T3)
        n190 = Generate User Event(user event=w796, event data cluster=w782) -> (user event out=w790:refnum<user-event>, error out=w789:errorcluster)  [unwired: 2 in]
        n191 = case shown="True" w786 {
          tunnel: w790 -> [_ w808]
          tunnel: w789 -> [_ w807]
          tunnel: w787 -> [w797 w799]
          tunnel: [w797 w799] -> w785
          tunnel: w784 -> [_ w804]
          frame False {
          }
          frame True {
            n192 = Empty String/Path?(string/path=w799) -> (empty?=w802:bool)
            n193 = Select(t="<Empty>" ("Current State"), s=w802, f=w799) -> (s? t:f=w801:string)
            n194 = Bundle By Name(cluster=T3 {"Name(\"\" to use uuid)"="", "Current State"="", "Arguments"="", "Argument - State"="", "From Who"="", "Complete(T)/Start(F)"=FALSE, "Type"=enum."State Change"} ("event data"), "Name(\"\" to use uuid)"=w804, "Current State"="<Remaining States>", "Arguments"=w801, "Type"=_JKISM_GlobalLog_MSG_TYPE."State Change") -> (w805:T3)
            n195 = Generate User Event(user event=w808, event data cluster=w805, error in=w807) -> ()  [unwired: 1 in, 2 out]
          }
        }
      }
      frame True {
      }
    }
    n196 = in-place-match #5(w771) -> (→"Name Used":string)
    n197 = in-place-match #6(w775) -> (→"Current State":string)
    n198 = in-place-match #7(w774) -> (→"Arguments":string)
    n199 = in-place-match #8(w773) -> (→"Argument - State":string)
    n200 = in-place-match #9(w772) -> (→"From Who":string)
    n201 = in-place-match #10(w769) -> (→"Remaining States":string)
  }
  n202 = feedback-in #1(w2) -> ()
